vi "AxisGoHome.vi"(8 "error in (no error)":errorcluster, 11 "DMC_1000B in":refnum<class "DMC_1000B.lvclass">) -> (0 "error out":errorcluster, 3 "DMC_1000B out":refnum<class "DMC_1000B.lvclass">)   [LabVIEW 2019, in "DMC_1000B.lvclass"]
uses:
  DMC_1000B.lvclass
  LLB/DMC1000B/Dmc1000/Dmc1000.lvlib
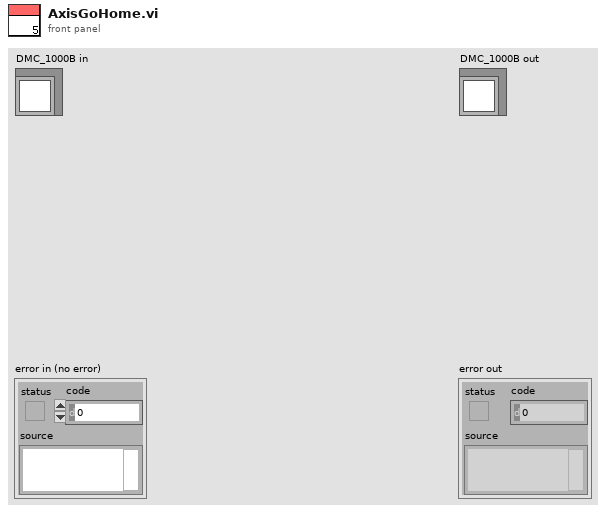
[diagram p1: front panel]
types:
  T1 = cluster{"AxisName":string, "Accel":dbl, "Deaccel":dbl, "Speed":dbl, "Sramp":dbl}[]
  T2 = cluster{"AxisName":string, "Accel":dbl, "Deaccel":dbl, "Speed":dbl, "Sramp":dbl}
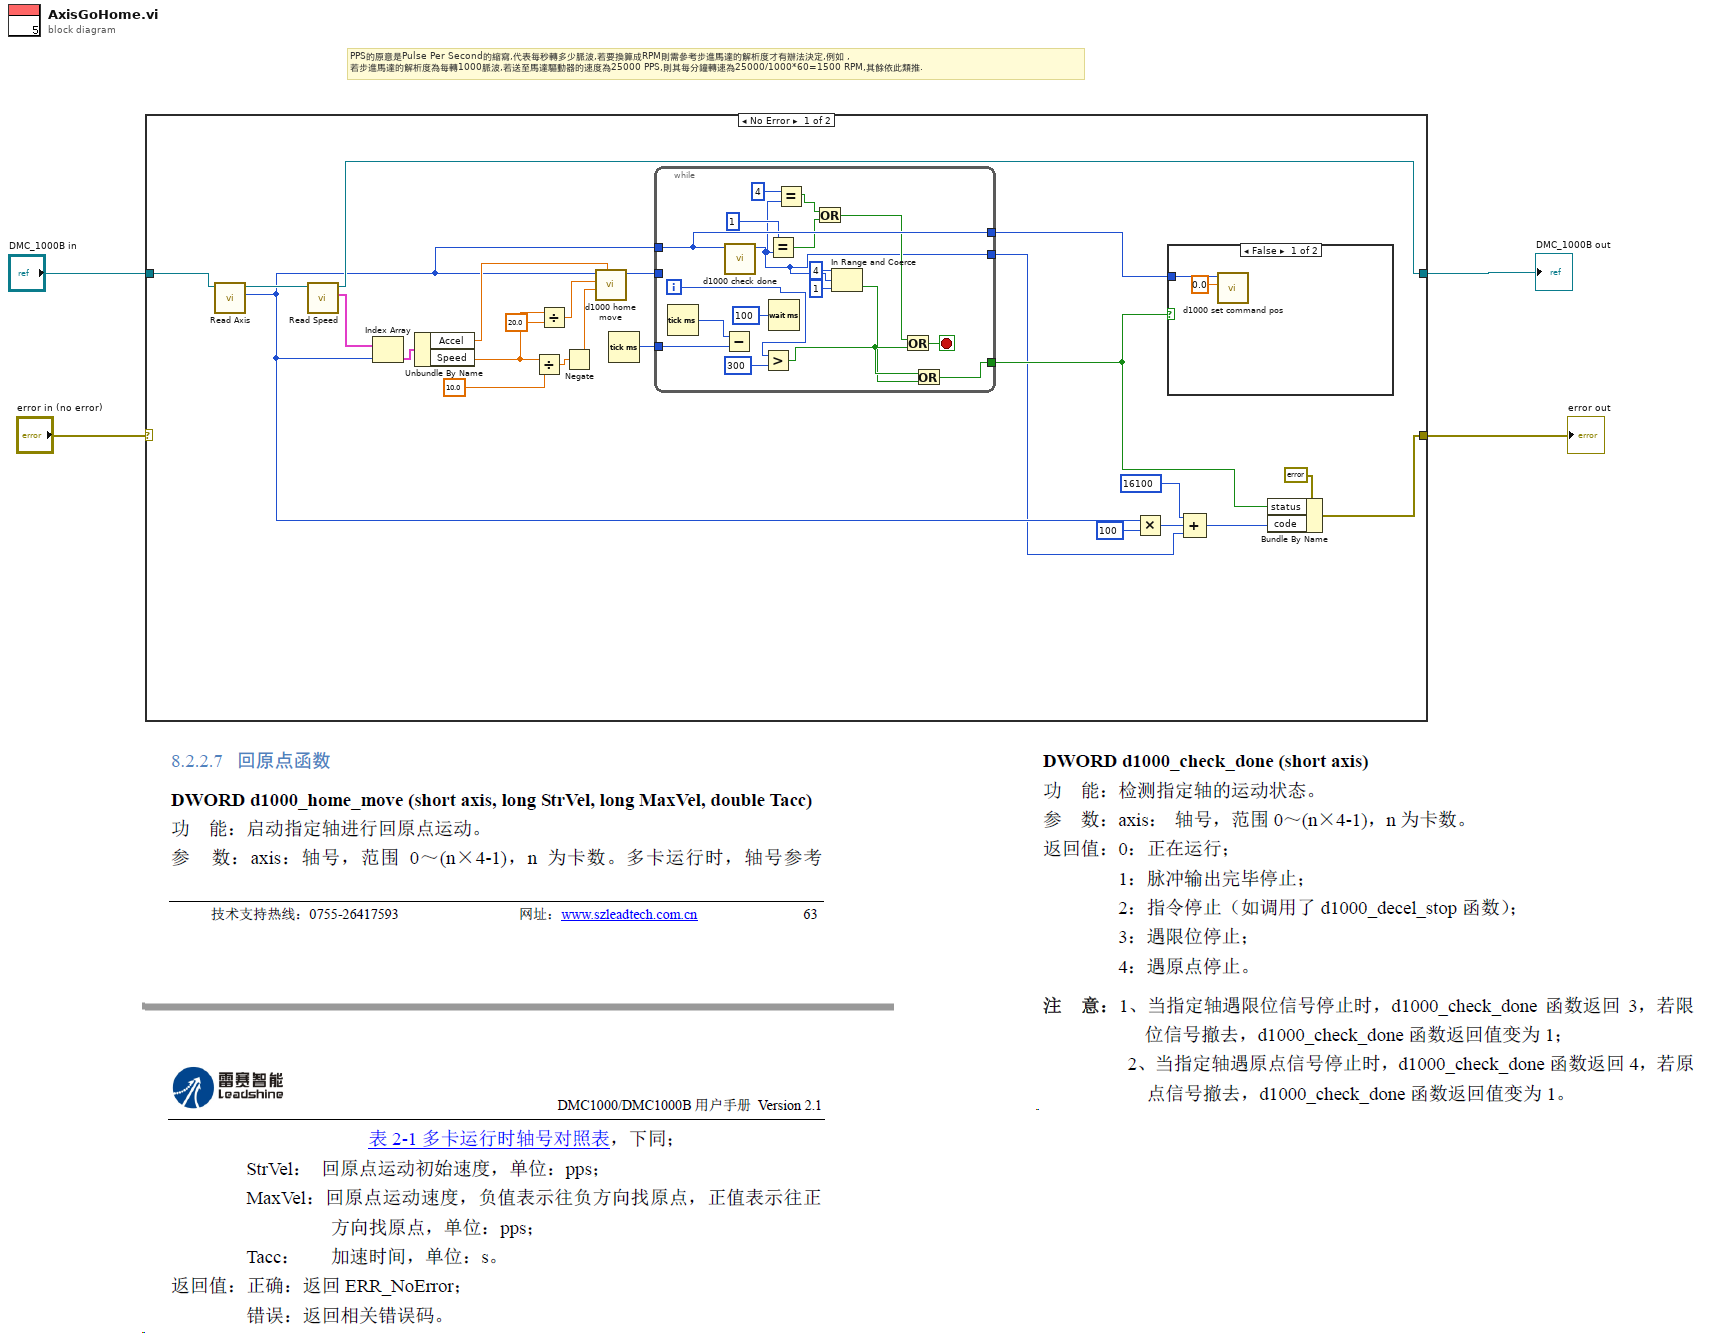
[diagram p0: block diagram]
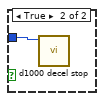
[diagram p2: hidden frame]
diagram:
  # "PPS的原意是Pulse Per Second的縮寫,代表每秒轉多少脈波,若要換算成RPM則需參考步進馬達的解析度才有辦法決定,例如 ,\n若步進馬達的解析度為每轉1000脈波,若送至馬達驅動器的速度為25000 PPS,則其每分鐘轉速為25000/1000*60=1500 RPM,其餘依此類推."
  n1 = case shown="No Error" "error in (no error)" {
    selector: "error in (no error)" -> [_ w51]
    tunnel: [w7 w51] -> w3
    tunnel: [w16 w50] -> w2
    tunnel: "DMC_1000B in" -> [w28 w50]
    frame No Error {
      n2 = call-dynamic "Read Axis.vi"("AxisCard in"=w28) -> ("Axis"=w11:u32, "AxisCard out"=w27:refnum<class "DMC_1000B.lvclass">)  [unwired: 8 in, 1 out]
      n3 = call-dynamic "Read Speed.vi"("AxisCard in"=w27) -> ("AxisSpeed"=w26:T1, "AxisCard out"=w16:refnum<class "DMC_1000B.lvclass">)  [unwired: 8 in, 1 out]
      n4 = Index Array(array=w26, index=w11) -> (element=w25:T2)
      n5 = Unbundle By Name(w25) -> ("Accel"=w19:dbl, "Speed"=w22:dbl)
      n6 = Divide(x=w22, y=10.0) -> (x/y=w23:dbl)
      n7 = Divide(x=w22, y=20.0) -> (x/y=w21:dbl)
      n8 = Negate(x=w23) -> (-x=w18:dbl)
      n9 = call "d1000 home move.vi"("Tacc"=w19, "MaxVel"=w18, "StrVel"=w21, "axis"=w11) -> ("function return"=w15:u32)  [unwired: 7 in]
      n10 = Tick Count (ms)() -> (millisecond timer value=w17:u32)
      n11 = while {
        tunnel: w11 -> [w45]
        tunnel: w17 -> [w47]
        tunnel: w15 -> [_]
        tunnel: [w45] -> w14
        tunnel: [w43] -> w6
        tunnel: [w34] -> w5
        i -> [w40]
        stop <- w44 stop-if-true
        n12 = Tick Count (ms)() -> (millisecond timer value=w48:u32)
        n13 = Subtract(x=w48, y=w47) -> ()  [unwired: 1 out]
        n14 = call "d1000 check done.vi"("axis"=w45) -> ("function return"=w34:u32)  [unwired: 10 in]
        n15 = Greater?(x=w40, y=u32 300) -> (0:w42:bool)
        n16 = Equal?(x=u32 1, y=w34) -> (x = y?=w38:bool)
        n17 = Wait (ms)(milliseconds to wait=u32 100) -> ()  [unwired: 1 out]
        n18 = Equal?(x=u32 4, y=w34) -> (x = y?=w37:bool)
        n19 = Or(x=w37, y=w38) -> (x .or. y?=w36:bool)
        n20 = In Range and Coerce(upper limit=u32 4, x=w34, lower limit=u32 1) -> (In Range?=w35:bool)  [unwired: 1 out]
        n21 = Or(x=w36, y=w42) -> (x .or. y?=w44:bool)
        n22 = Or(x=w42, y=w35) -> (x .or. y?=w43:bool)
      }
      n23 = Multiply(x=w11, y=u32 100) -> (x*y=w12:u32)
      n24 = case shown="False" w6 {
        tunnel: w14 -> [w30 w31]
        frame False {
          n25 = call "d1000 set command pos.vi"("Pos"=0.0, "axis"=w30) -> ()  [unwired: 9 in, 1 out]
        }
        frame True {
          n26 = call "d1000 decel stop.vi"("axis"=w31) -> ()  [unwired: 10 in, 1 out]
        }
      }
      n27 = Compound Arithmetic op=ADD(16100, w12, w5) -> (w8:u32)
      n28 = Bundle By Name(cluster=errorcluster {"status"=FALSE, "code"=0, "source"=""} ("error constant"), "status"=w6, "code"=w8) -> (w7:errorcluster)
    }
    frame Error {
    }
  }
  "error out" <- w3
  "DMC_1000B out" <- w2
